vi "Write Voltage Actual (Single).vi"(8 "error in":errorcluster, 9 "Channel Index":i32=1, 10 "Voltage":dbl, 11 "Cycler in":refnum<class "Cycler.lvclass">) -> (0 "error out":errorcluster, 3 "Cycler out":refnum<class "Cycler.lvclass">)   [LabVIEW 2023, in "Cycler.lvclass"]
uses:
  Cycler.lvclass
  Cycler.lvclass/Cycler.ctl
  <vilib>/ADAS Replay HIL/Channels/Tag Wrapper/Tag Wrapper.lvlib
  <vilib>/ADAS Replay HIL/Channels/Tag Wrapper/Polymorphic/Write Channel (Double).vi
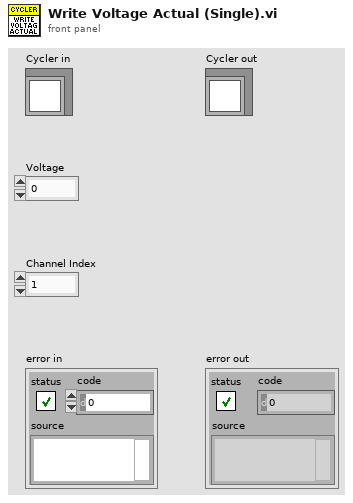
[diagram p1: front panel]
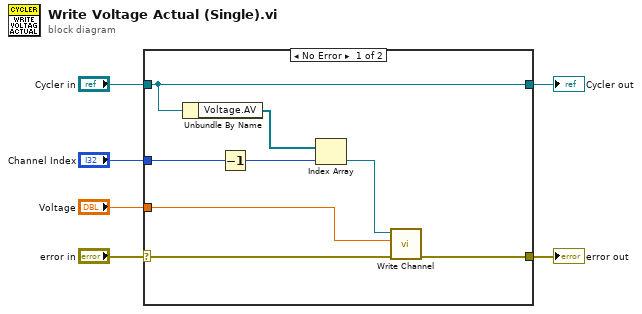
[diagram p0: block diagram]
diagram:
  n1 = case shown="No Error" "error in" {
    selector: "error in" -> [w14 w15]
    tunnel: [w13 w15] -> w5
    tunnel: [w11 w16] -> w3
    tunnel: "Cycler in" -> [w11 w16]
    tunnel: "Voltage" -> [w12 _]
    tunnel: "Channel Index" -> [w8 _]
    frame No Error {
      n2 = Unbundle By Name(w11) -> ("Voltage.AV"=w10:refnum<k21>[])
      n3 = Decrement(x=w8) -> (x-1=w7:i32)
      n4 = Index Array(array=w10, index=w7) -> (element=w9:refnum<k21>)
      n5 = call-poly <vilib>:"Write Channel.vi"("error in"=w14, "Value to Write"=w12, "ADAS HIL Channel in"=w9) -> ("error out"=w13:errorcluster)  [unwired: 6 in, 2 out]
    }
    frame Error {
    }
  }
  "error out" <- w5
  "Cycler out" <- w3
